vi "Write Chapter.vi"(0 "PDF Report Class in":refnum<class "PDF Report Class.lvclass">, 7 "Chapter ref":T1, 11 "error in (no error)":errorcluster) -> (4 "PDF Report Class out":refnum<class "PDF Report Class.lvclass">, 15 "error out":errorcluster)   [LabVIEW 2019, in "Exaprom PDF.lvlib" / "PDF Report Class.lvclass"]
uses:
  PDF Report Class.lvclass
  C:/work/niobrara_lv/labview pdf writer fixing/DLL/itextsharp.dll
  DLL/itextsharp.dll
  PDF Report Class.lvclass/PDF Report Class.ctl
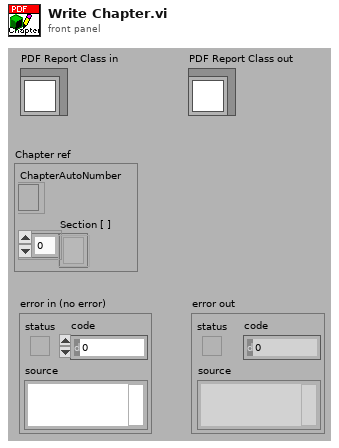
[diagram p1: front panel]
types:
  T1 = cluster{"ChapterAutoNumber":refnum<k24>, "Section [ ]":refnum<k24>[]}
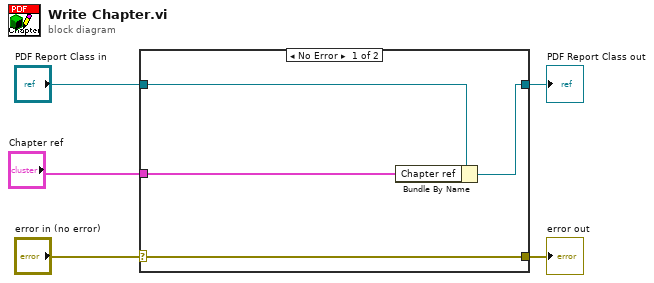
[diagram p0: block diagram]
diagram:
  n1 = case shown="No Error" "error in (no error)" {
    selector: "error in (no error)" -> [w9 w10]
    tunnel: [w9 w10] -> w4
    tunnel: [w7 w11] -> w2
    tunnel: "PDF Report Class in" -> [w8 w11]
    tunnel: "Chapter ref" -> [w6 _]
    frame No Error {
      n2 = Bundle By Name(cluster=w8, "Chapter ref"=w6) -> (w7:refnum<class "PDF Report Class.lvclass">)
    }
    frame Error {
    }
  }
  "error out" <- w4
  "PDF Report Class out" <- w2
